vi "RESTful Buffer Mode To Text.vi"(1 "Buffer Mode":bool) -> (0 "Boolean Text":string)   [LabVIEW 2020]
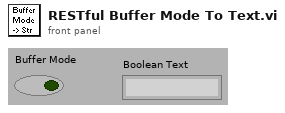
[diagram p1: front panel]
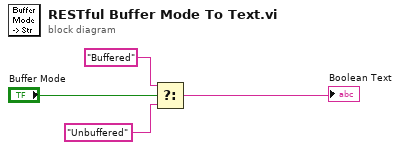
[diagram p0: block diagram]
diagram:
  n1 = Select(t="Buffered", s="Buffer Mode", f="Unbuffered") -> (s? t:f=→"Boolean Text":string)
